vi "Withdraw Amount.vi"(10 "User Input":string, 11 "Module Data in":T1) -> (2 "Withdrawal Complete Message":string, 3 "Module Data out":T1)   [LabVIEW 2016]
doc: "Check if account has sufficient funds"
uses:
  <vilib>/Utility/file.llb/Write Delimited Spreadsheet (string).vi
  Controls/UI Controls.ctl
  Controls/ATM Messages.ctl
  Controls/Transaction Status.ctl
  Controls/User Input Data.ctl
  Controls/Module Data.ctl
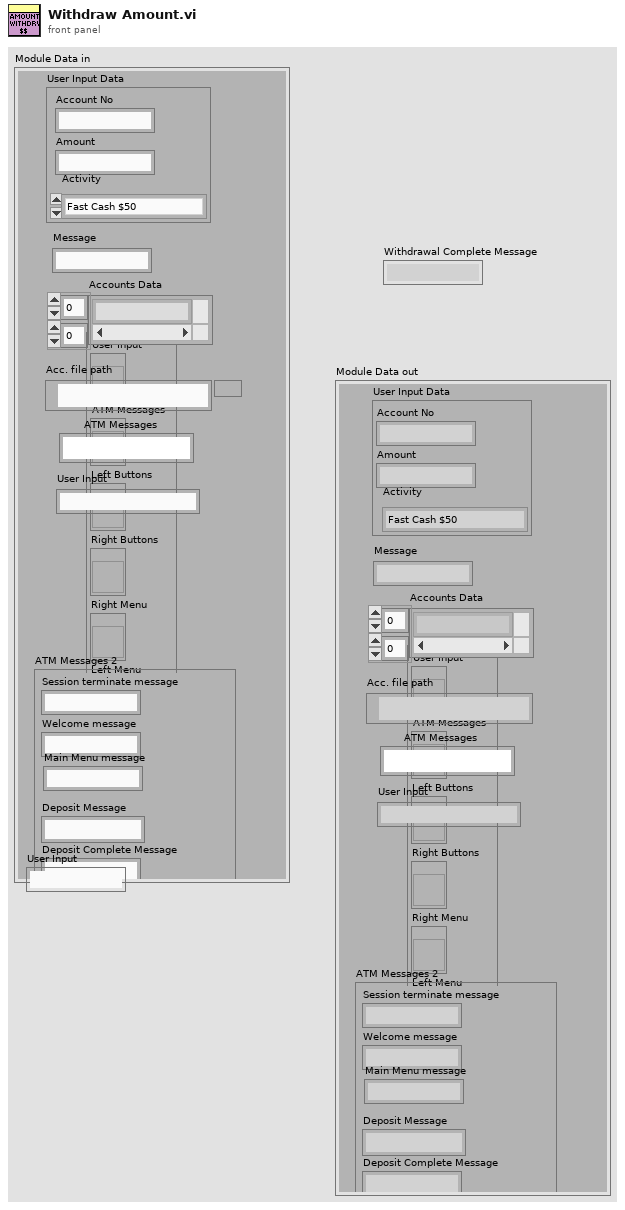
[diagram p1: front panel]
types:
  T1 = typedef "Module Data.ctl" = cluster{"UI Controls":T2, "ATM Messages 2":T3, "User Input":string, "ATM Messages":string, "Acc. file path":path, "Accounts Data":string[][], "User Input Data":T4, "Message":string}
  T2 = typedef "UI Controls.ctl" = cluster{"ATM Messages":refnum<vi>, "User Input":refnum<vi>, "Right Buttons":refnum<vi>, "Right Menu":refnum<vi>, "Left Buttons":refnum<vi>, "Left Menu":refnum<vi>, "Card Simulator":refnum<vi>, "Enter":refnum<vi>}
  T3 = typedef "ATM Messages.ctl" = cluster{"Session terminate message":string, "Welcome message":string, "Deposit Message":string, "Deposit Complete Message":string, "Withdrawal Message":string, "Withdrawal Complete Message":string, "Balance Inquiry Message":string, "Account verification failed message":string, "Withdrawal failed message":string, "Card Inserted":string, "Main Menu message":string}
  T4 = typedef "User Input Data.ctl" = cluster{"Account No":string, "Amount":string, "Activity":T5}
  T5 = typedef "Transaction Status.ctl" = enum16{"Fast Cash $50", "Withdrawal?", "Deposit?", "Account Number?"}
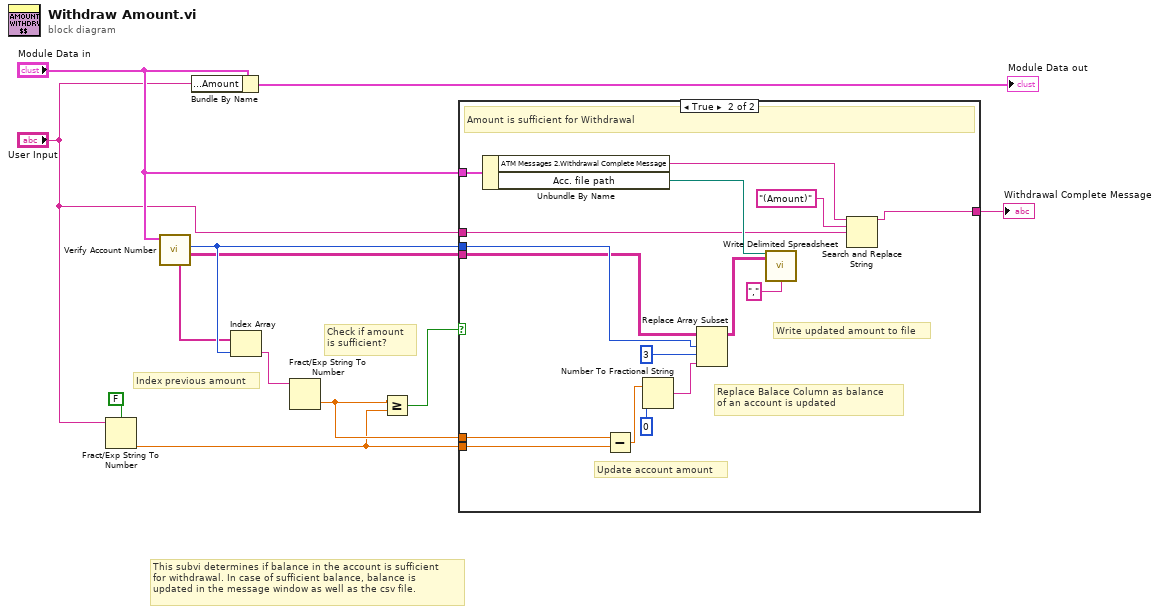
[diagram p0: block diagram]
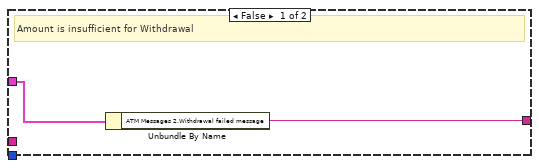
[diagram p2: hidden frame]
diagram:
  # "This subvi determines if balance in the account is sufficient\nfor withdrawal. In case of sufficient balance, balance is \nupdated in the message window as well as the csv file."
  # "Check if amount\nis sufficient?"
  # "Index previous amount"
  n1 = Fract/Exp String To Number(use system decimal point (T)=FALSE, string="User Input") -> (number=w3:dbl)  [unwired: 2 in, 1 out]
  n2 = call "Verify Account Number.vi"("Module Data"="Module Data in") -> ("Accounts all data"=w7:string[][], "Index account no."=w8:i32, "Balances Column"=w6:string[])  [unwired: 6 in, 2 out]
  n3 = Bundle By Name(cluster="Module Data in", "User Input Data.Amount"="User Input") -> (→"Module Data out":T1)
  n4 = Index Array(array=w6, index=w8) -> (element=w11:string)
  n5 = Fract/Exp String To Number(string=w11) -> (number=w4:dbl)  [unwired: 3 in, 1 out]
  n6 = Greater Or Equal?(x=w4, y=w3) -> (x >= y?=w2:bool)
  n7 = case shown="True" w2 {
    tunnel: "Module Data in" -> [w14 w29]
    tunnel: w8 -> [_ w28]
    tunnel: w7 -> [_ w23]
    tunnel: "User Input" -> [_ w18]
    tunnel: w4 -> [_ w17]
    tunnel: w3 -> [_ w16]
    tunnel: [w13 w15] -> w1
    frame False {
      # "Amount is insufficient for Withdrawal"
      n8 = Unbundle By Name(w14) -> ("ATM Messages 2.Withdrawal failed message"=w13:string)
    }
    frame True {
      # "Write updated amount to file"
      # "Update account amount"
      # "Replace Balace Column as balance \nof an account is updated"
      # "Amount is sufficient for Withdrawal"
      n9 = Unbundle By Name(w29) -> ("ATM Messages 2.Withdrawal Complete Message"=w19:string, "Acc. file path"=w24:path)
      n10 = Subtract(x=w17, y=w16) -> (x-y=w30:dbl)
      n11 = Number To Fractional String(number=w30, precision (6)=i16 0) -> (F-format string=w21:string)  [unwired: 2 in]
      n12 = Replace Array Subset(array=w23, new element=w21, index (row)=w28, index (col)=3 ("disabled index (col)")) -> (w27:string[][])
      n13 = call-poly <vilib>:"Write Delimited Spreadsheet.vi"("file path (dialog if empty)"=w24, "2D data"=w27, "delimiter (\\t)"="," ("delimiter (\\t)")) -> ()  [unwired: 11 in, 2 out]
      n14 = Search and Replace String(input string=w19, search string="(Amount)" ("search string/char (-)"), replace string=w18) -> (result string=w15:string)  [unwired: 5 in, 3 out]
    }
  }
  "Withdrawal Complete Message" <- w1
